vi "monochromatorCommandSetFilterLabel.vi"(8 "error in":errorcluster, 9 "label":string, 10 "filter_position":i32, 11 "monochromator":refnum<k24>) -> (0 "error out":errorcluster, 3 "monochromator":refnum<k24>)   [LabVIEW 2009]
doc: "Set filter label for a requested filter"
uses:
  C:/Users/anderson.chen/Desktop/Software Development/Cornerstone Series API (LV9)/Cornerstone DLL/Cornerstone.dll
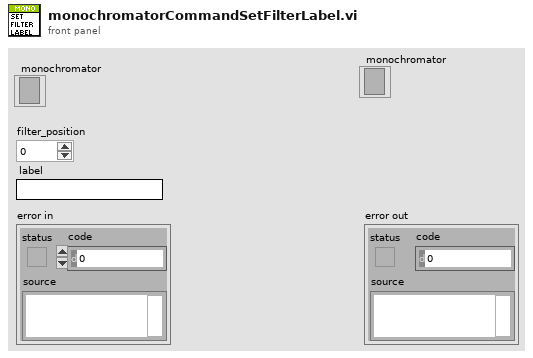
[diagram p1: front panel]
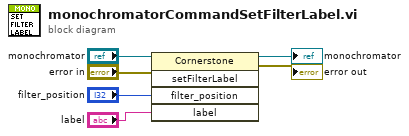
[diagram p0: block diagram]
diagram:
  n1 = invoke class="Cornerstone" method="setFilterLabel"(reference="monochromator", error in="error in", "filter_position"="filter_position", "label"="label") -> (reference out=→"monochromator":refnum<k24>, error out=→"error out":errorcluster)  [unwired: 1 in, 3 out]
